vi "CheckForAlerts.vi"(8 "error in (no error)":errorcluster, 11 "Axis in":refnum<class "Axis.lvclass">) -> (0 "error out":errorcluster, 1 "ToString":string, 2 "Boolean":bool, 3 "Axis out":refnum<class "Axis.lvclass">)   [LabVIEW 2020, in "Axis.lvclass"]
uses:
  Axis.lvclass
  Axis.lvclass/Axis.ctl
  C:/Users/Jonathan/Documents/Clearpath SDK/CSharp Examples/CLRWrapper/x64/Debug/CLRWrapper.dll
  CSharp Examples/CLRWrapper/x64/Debug/CLRWrapper.dll
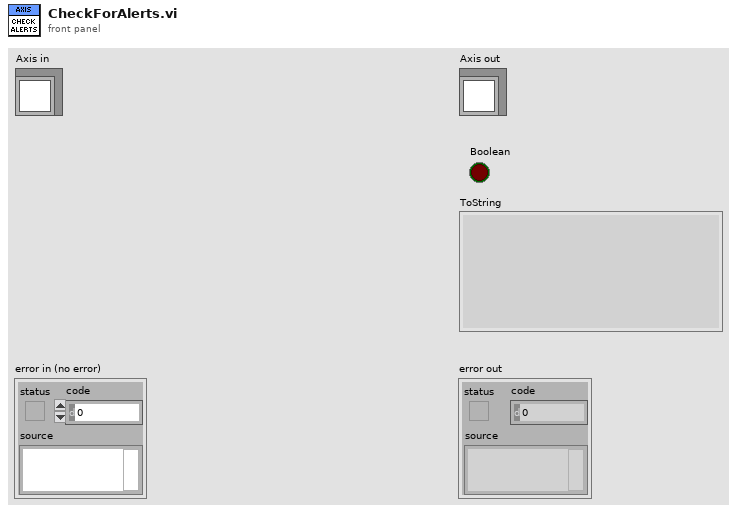
[diagram p1: front panel]
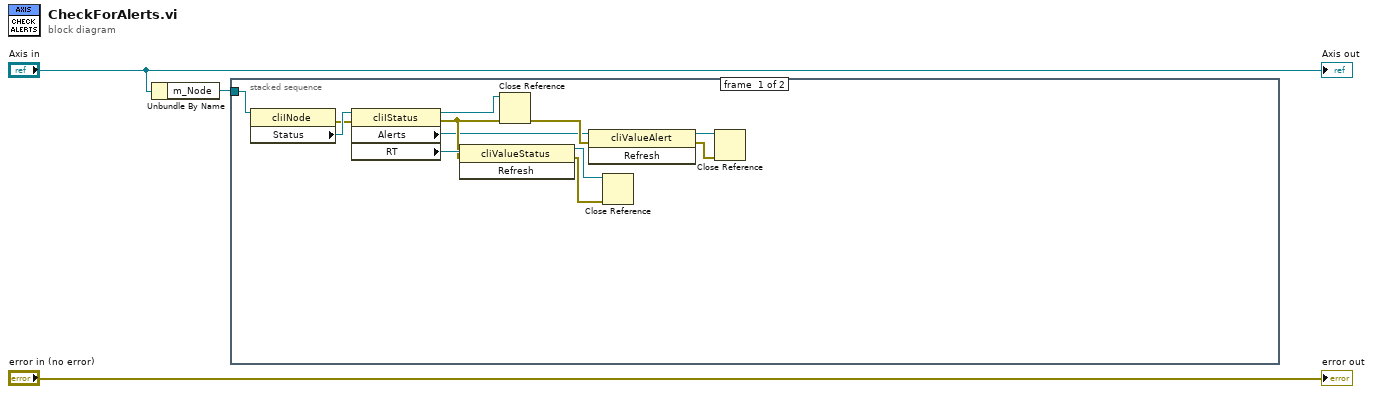
[diagram p0: block diagram]
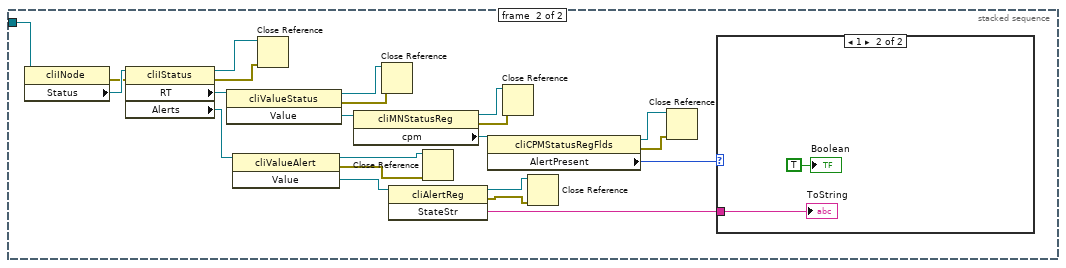
[diagram p2: hidden frame]
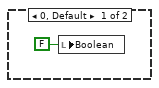
[diagram p3: hidden frame]
diagram:
  n1 = Unbundle By Name("Axis in") -> ("m_Node"=w1:refnum<k24>)
  n2 = stacked-sequence {
    tunnel: w1 -> [w15 w37]
    frame #0 {
      n3 = property class="cliINode"(reference=w15) -> (error out=w4:errorcluster, "Status"=w14:refnum<k24>)  [unwired: 1 in, 1 out]
      n4 = property class="cliIStatus"(reference=w14, error in=w4) -> (reference out=w12:refnum<k24>, error out=w7:errorcluster, "Alerts"=w5:refnum<k24>, "RT"=w13:refnum<k24>)
      n5 = invoke class="cliValueStatus" method="Refresh"(reference=w13, error in=w7) -> (reference out=w9:refnum<k24>, error out=w8:errorcluster)  [unwired: 1 in, 1 out]
      n6 = Close Reference(reference=w12, error in (no error)=w7) -> (error out=w6:errorcluster)
      n7 = invoke class="cliValueAlert" method="Refresh"(reference=w5, error in=w6) -> (reference out=w10:refnum<k24>, error out=w11:errorcluster)  [unwired: 1 in, 1 out]
      n8 = Close Reference(reference=w9, error in (no error)=w8) -> ()  [unwired: 1 out]
      n9 = Close Reference(reference=w10, error in (no error)=w11) -> ()  [unwired: 1 out]
    }
    frame #1 {
      n10 = property class="cliINode"(reference=w37) -> (error out=w35:errorcluster, "Status"=w36:refnum<k24>)  [unwired: 1 in, 1 out]
      n11 = property class="cliIStatus"(reference=w36, error in=w35) -> (reference out=w31:refnum<k24>, error out=w29:errorcluster, "RT"=w34:refnum<k24>, "Alerts"=w22:refnum<k24>)
      n12 = invoke class="cliValueStatus" method="Value"(reference=w34) -> (reference out=w30:refnum<k24>, error out=w28:errorcluster, "Value"=w33:refnum<k24>)  [unwired: 2 in]
      n13 = invoke class="cliValueAlert" method="Value"(reference=w22) -> (reference out=w17:refnum<k24>, error out=w16:errorcluster, "Value"=w21:refnum<k24>)  [unwired: 2 in]
      n14 = Close Reference(reference=w31, error in (no error)=w29) -> ()  [unwired: 1 out]
      n15 = property class="cliMNStatusReg"(reference=w33) -> (reference out=w27:refnum<k24>, error out=w26:errorcluster, "cpm"=w32:refnum<k24>)  [unwired: 1 in]
      n16 = Close Reference(reference=w30, error in (no error)=w28) -> ()  [unwired: 1 out]
      n17 = invoke class="cliAlertReg" method="StateStr"(reference=w21) -> (reference out=w19:refnum<k24>, error out=w18:errorcluster, "StateStr"=w20:string)  [unwired: 2 in]
      n18 = Close Reference(reference=w17, error in (no error)=w16) -> ()  [unwired: 1 out]
      n19 = property class="cliCPMStatusRegFlds"(reference=w32) -> (reference out=w24:refnum<k24>, error out=w25:errorcluster, "AlertPresent"=w23:u16)  [unwired: 1 in]
      n20 = Close Reference(reference=w27, error in (no error)=w26) -> ()  [unwired: 1 out]
      n21 = Close Reference(reference=w19, error in (no error)=w18) -> ()  [unwired: 1 out]
      n22 = Close Reference(reference=w24, error in (no error)=w25) -> ()  [unwired: 1 out]
      n23 = case shown="1" w23 {
        tunnel: w20 -> [_ w40]
        frame 0, Default {
          n24 = local write "Boolean"(FALSE ("Boolean")) -> ()
        }
        frame 1 {
          "ToString" <- w40
          "Boolean" <- TRUE ("Boolean")
        }
      }
    }
  }
  "error out" <- "error in (no error)"
  "Axis out" <- "Axis in"
